vi "Model Initial Values - Global.vi"() -> ()   [LabVIEW 2011, in "Model Initial Values Custom Device.lvlib"]
uses:
  Model Initial Values Custom Device.lvlib
panel:
  in  "Model Num Inports":string="Model Num Inports"
  in  "Model Checksum":string="Model Checksum"
  in  "Inport Default Values":string="Inport Default Values"
  in  "Inport Names":string="Inport Names"
  in  "Export Dynamic Btn":string="NIVS_InitValues_Export"
  in  "Remove Dynamic Btn":string="NIVS_InitValues_RemoveModels"
  in  "Model Names":string="Model Names"
  in  "Inport References":string="Inport References"
  in  "Model Reference":string="Model Reference"
  in  "Model Page GUID":string="806F417C-F0ED-C4A2-47CB-356CC3490174"
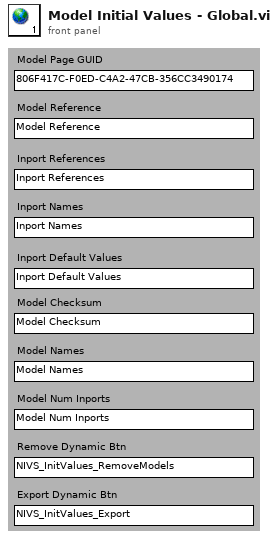
[diagram p1: front panel]
diagram:
